vi "Read All Elements GUI.vi"(8 "error in (no error)":errorcluster, 11 "Config params in":refnum<class "CV-Configuration.lvclass">) -> (0 "error out":errorcluster, 2 "Configuration params.":T1={"Number of cameras"=1, "Camera 1 port"=enum."B", "ROI width"=0, "ROI height"=1248, "Reset ROI"=FALSE, "Width scale"=0.05, "Height scale"=0.05, "Center Y cam. 1"=0, "Center X cam. 1"=541, "Center Y cam. 2"=624, "Center X cam. 2"=541} {"Center X cam. 2" min=4 max=1244 step=8; "Center Y cam. 2" min=1 max=1082 step=1; "Center X cam. 1" min=4 max=1244 step=8; "Center Y cam. 1" min=1 max=1082 step=1; "Height scale" min=0.001 step=0.001 format="%.3f"; "Width scale" min=0.001 step=0.001 format="%.3f"; "Number of cameras" min=1 max=2 step=1; "ROI width" min=8 max=1248 step=8; "ROI height" min=1 max=1082 step=1}, 3 "Config params out":refnum<class "CV-Configuration.lvclass">)   [LabVIEW 2013, in "CameraVision.lvlib" / "CV-Configuration.lvclass"]
uses:
  CV-Configuration.lvclass
  Configuration-parameters-gui.ctl
  CV-Configuration.lvclass/CV-Configuration.ctl
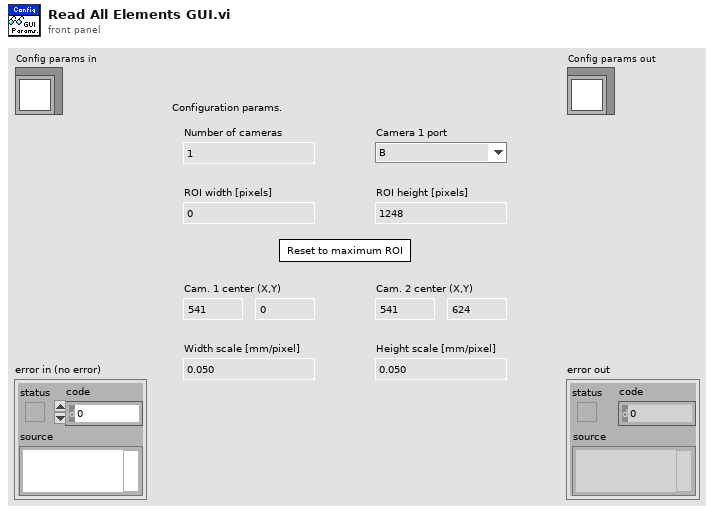
[diagram p1: front panel]
types:
  T1 = typedef "CameraVision.lvlib/CV-Configuration.lvclass/Configuration-parameters-gui.ctl" = cluster{"Number of cameras":i32, "Camera 1 port":enum16{"A", "B"}, "ROI width":u32, "ROI height":u32, "Reset ROI":bool, "Width scale":dbl, "Height scale":dbl, "Center Y cam. 1":i32, "Center X cam. 1":i32, "Center Y cam. 2":i32, "Center X cam. 2":i32}
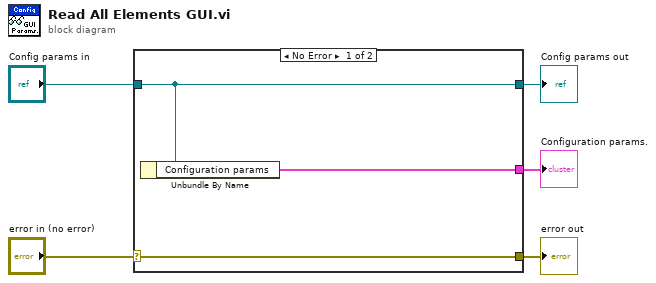
[diagram p0: block diagram]
diagram:
  n1 = case shown="No Error" "error in (no error)" {
    selector: "error in (no error)" -> [w8 w9]
    tunnel: [w8 w9] -> w4
    tunnel: [w7 w10] -> w2
    tunnel: "Config params in" -> [w7 w10]
    tunnel: [w6 _] -> w1
    frame No Error {
      n2 = Unbundle By Name(w7) -> ("Configuration params"=w6:T1)
    }
    frame Error {
    }
  }
  "error out" <- w4
  "Config params out" <- w2
  "Configuration params." <- w1
